vi "CloseAppRefInClusterArray.vi"(1 "Array":cluster{"App Refnum":refnum<vi>}[](array[cluster])) -> (0 "error out":errorcluster)   [LabVIEW 2011]
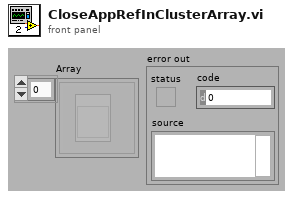
[diagram p1: front panel]
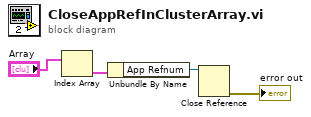
[diagram p0: block diagram]
diagram:
  n1 = Index Array(array="Array") -> (element=w2:cluster{"App Refnum":refnum<vi>})  [unwired: 1 in]
  n2 = Unbundle By Name(w2) -> ("App Refnum"=w1:refnum<vi>)
  n3 = Close Reference(reference=w1) -> (error out=→"error out":errorcluster)  [unwired: 1 in]
